vi "Save BG Image.vi"(8 "error in (no error)":errorcluster, 11 "HIJ Vision Camera App In":refnum<class "HIJ Vision Camera App.lvclass">) -> (0 "error out":errorcluster, 2 "image path":path, 3 "HIJ Vision Camera App Out":refnum<class "HIJ Vision Camera App.lvclass">)   [LabVIEW 2020, in "HIJ Vision Camera App.lvlib" / "HIJ Vision Camera App.lvclass"]
doc: "Speichert das Kamerabild in PNG Format und ruft Generate Report auf. Wenn Flag \"Time in Filename\" gesetzt ist, wird ein Zeitstempel dem Dateinamen angehängt."
uses:
  HIJ Vision Camera App.lvclass
  C:/Users/AlexK/work/LabVIEW Programme/POLARIS CAM Log Abw und E/Submodules/HIJ Vision/Application Base Actors/HIJ Vision Application/HIJ Vision Application/HIJ Vision Application.lvclass
  HIJ Vision Application/HIJ Vision Application/HIJ Vision Application.lvclass/HIJ Vision Application.ctl
  HIJ Vision Application/HIJ Vision Application/Read Raw Image.vi
  HIJ Vision Application/HIJ Vision Application/Read WorkDir.vi
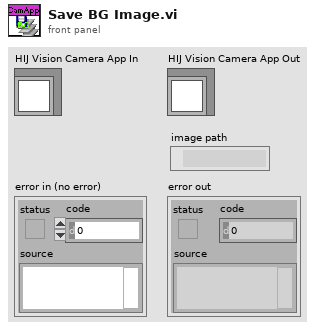
[diagram p1: front panel]
types:
  T1 = typedef "IMAQ Image.ctl" = refnum<image>
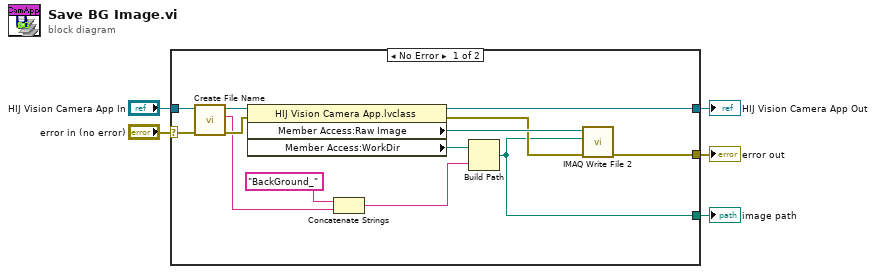
[diagram p0: block diagram]
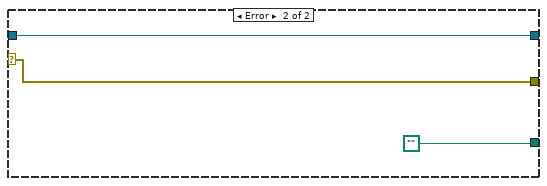
[diagram p2: hidden frame]
diagram:
  n1 = case shown="No Error" "error in (no error)" {
    selector: "error in (no error)" -> [w9 w21]
    tunnel: [w15 w21] -> w4
    tunnel: [w13 w20] -> w2
    tunnel: "HIJ Vision Camera App In" -> [w18 w20]
    tunnel: [w12 path ""] -> w1
    frame No Error {
      n2 = call-dynamic "Create File Name.vi"("error in (no error)"=w9, "HIJ Vision Camera App in"=w18) -> ("error out"=w10:errorcluster, "FileName"=w8:string, "HIJ Vision Camera App out"=w11:refnum<class "HIJ Vision Camera App.lvclass">)  [unwired: 7 in]
      n3 = property class="HIJ Vision Camera App.lvclass"(reference=w11, error in=w10) -> (reference out=w13:refnum<class "HIJ Vision Camera App.lvclass">, error out=w14:errorcluster, "Member Access:Raw Image"=w17:T1, "Member Access:WorkDir"=w16:path)
      n4 = Concatenate Strings("BackGround_" ("string"), w8) -> (w7:string)
      n5 = Build Path(base path=w16, name or relative path=w7) -> (appended path=w12:path)
      n6 = call-poly "IMAQ Write File 2"("error in (no error)"=w14, "File Path"=w12, "Image"=w17) -> ("error out"=w15:errorcluster)  [unwired: 7 in, 1 out]
    }
    frame Error {
    }
  }
  "error out" <- w4
  "HIJ Vision Camera App Out" <- w2
  "image path" <- w1
